vi "pwm_out.vi"(0 "pwm info":T1={"sample mode"=10178, "initial delay"=0.0, "idle state"=10214, "counter"="Dev1/ctr0", "channel name"="pwm out", "low time"=0.01, "high time"=0.01, "units"=10364, "number of samples"=100} {"sample mode" items=["Finite Samples"=10178, "Continuous Samples"=10123, "Hardware Timed Single Point"=12522]; "idle state" items=["High"=10192, "Low"=10214]; "units" items=["Seconds"=10364, "From Custom Scale"=10065]}, 11 "error in":errorcluster caption="错误输入") -> (15 "error out":errorcluster caption="错误输出")   [LabVIEW 2013]
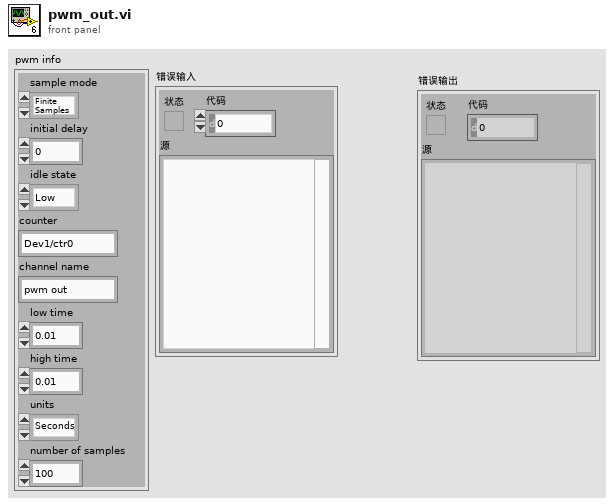
[diagram p1: front panel]
types:
  T1 = cluster{"sample mode":i32, "initial delay":dbl, "idle state":i32, "counter":string, "channel name":string, "low time":dbl, "high time":dbl, "units":i32, "number of samples":i32}
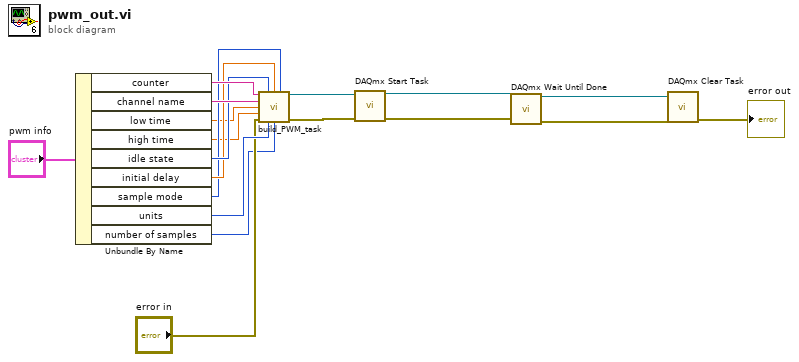
[diagram p0: block diagram]
diagram:
  n1 = Unbundle By Name("pwm info") -> ("counter"=w15:string, "channel name"=w14:string, "low time"=w7:dbl, "high time"=w6:dbl, "idle state"=w13:i32, "initial delay"=w12:dbl, "sample mode"=w11:i32, "units"=w10:i32, "number of samples"=w5:i32)
  n2 = call "build_PWM_task.vi"("counter"=w15, "idle state"=w13, "initial delay"=w12, "sample mode"=w11, "channel name"=w14, "low time"=w7, "high time"=w6, "error in"="error in", "units"=w10, "number of samples"=w5) -> ("task out"=w8:refnum<k21>, "error out"=w18:errorcluster)  [unwired: 4 in]
  n3 = call <vilib>:"DAQmx Start Task.vi"("task/channels in"=w8, "error in"=w18) -> ("task out"=w4:refnum<k21>, "error out"=w3:errorcluster)  [unwired: 12 in]
  n4 = call <vilib>:"DAQmx Wait Until Done.vi"("task/channels in"=w4, "error in"=w3) -> ("task out"=w2:refnum<k21>, "error out"=w1:errorcluster)  [unwired: 12 in]
  n5 = call <vilib>:"DAQmx Clear Task.vi"("task in"=w2, "error in"=w1) -> ("error out"=→"error out":errorcluster)  [unwired: 13 in]
